vi "Deserialize Data.vi"(8 "error in (no error)":errorcluster, 11 "Flat Data in":string) -> (0 "error out":errorcluster, 3 "Process Data out":T1)   [LabVIEW 2020, in "Waveform(DBL) Array.lvlib"]
doc: "Version 0.1"
uses:
  <vilib>/ADAS Record/CustomDataTypes/Waveform(DBL) Array/Waveform(DBL) Array.lvlib
  <vilib>/ADAS Record/CustomDataTypes/Waveform(DBL) Array/Process Data.ctl
  <vilib>/ADAS Record/IODataPEF/CfgMgr/FlatFormat.ctl
  5e2451cd-7b8c-4079-9add-41a600a01e16.vi
  <vilib>/ADAS Record/IODataPEF/Error/Error_SetError.vi
  <vilib>/ADAS Record/IODataPEF/Error/Error_CheckAndSetDllError.vi
  <vilib>/ADAS Record/IODataPEF/Error/ErrorMgr.vi
  <vilib>/ADAS Record/CustomData/_Custom_RegisterType.vi
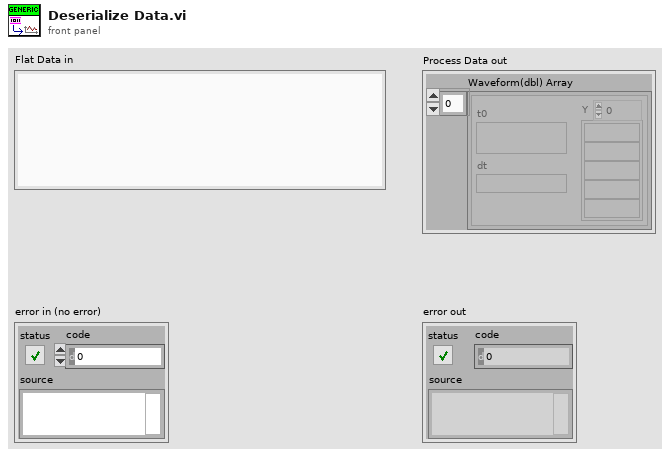
[diagram p1: front panel]
types:
  T1 = typedef "Waveform(DBL) Array.lvlib/Process Data.ctl" = cluster{"Waveform(dbl) Array":waveform(dbl)[]}
  T2 = typedef "FlatFormat.ctl" = enum32{"Auto", "PEF", "GFB (Apache)", "GFB", "JSON", "Readable JSON", "LV String", "Reserved", "LV Native"}
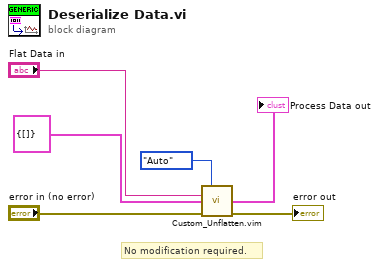
[diagram p0: block diagram]
diagram:
  # "No modification required."
  n1 = call "Custom_Unflatten.vim"("Flat Format"=FlatFormat."Auto", "Flat Data"="Flat Data in", "Data (type/default value)"=T1 {"Waveform(dbl) Array"=[]} ("Byte Array in"), "error in (no error)"="error in (no error)") -> ("Data"=→"Process Data out":T1, "Error (out)"=→"error out":errorcluster)  [unwired: 10 in]
